vi "TDK电流加载.vi"(5 "all rows":dbl[][](array[numeric]), 6 "停止":bool, 7 "电源台数":dbl=1.0, 8 "循环次数":i32, 9 "error out":errorcluster, 10 "Globalize (0: Single)":u16, 11 "VISA resource name out":refnum<visa-resource-name>) -> (1 "已完成循环次数":i32, 2 "error out 2":errorcluster caption="error out", 3 "VISA resource name out 2":refnum<visa-resource-name>)   [LabVIEW 2021]
uses:
  <instrlib>/TDK-Lambda G Series/TDK-Lambda G Series.lvlib
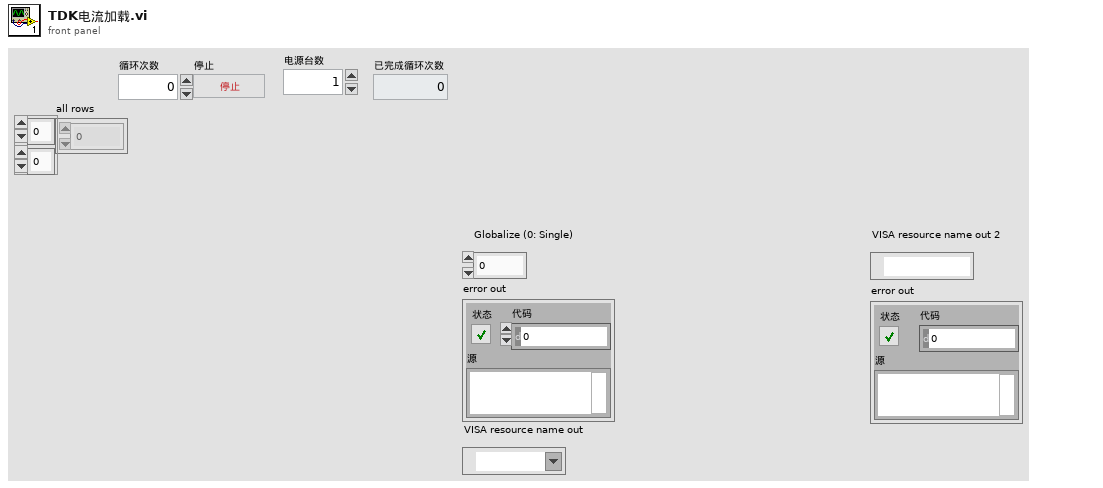
[diagram p1: front panel]
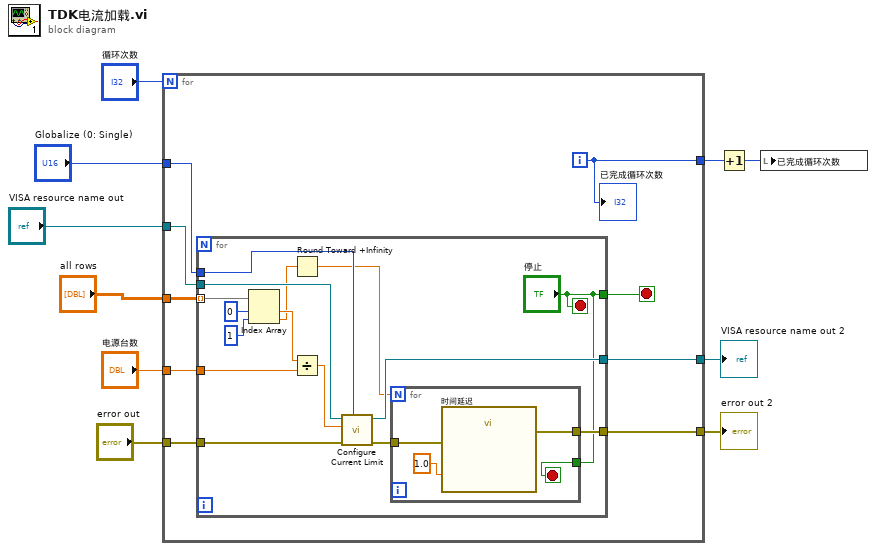
[diagram p0: block diagram]
diagram:
  n1 = for {
    N: "循环次数" -> [_]
    tunnel: "all rows" -> [w17]
    tunnel: "Globalize (0: Single)" -> [w16]
    tunnel: [w15] -> w9
    tunnel: "电源台数" -> [w14]
    tunnel: "error out" -> [w18]
    tunnel: [w11] -> w2
    tunnel: "VISA resource name out" -> [w19]
    tunnel: [w12] -> w3
    i -> [w15]
    stop <- w13 stop-if-true
    n2 = for {
      tunnel: w17 -> [w34] mode=indexing
      tunnel: w19 -> [w31]
      tunnel: w18 -> [w30]
      tunnel: [w28] -> w11
      tunnel: [w27] -> w12
      tunnel: w16 -> [w26]
      tunnel: w14 -> [w23]
      tunnel: ["停止"] -> w13
      stop <- "停止" stop-if-true
      n3 = Index Array(array=w34, index #1=0 ("索引"), index #2=1 ("索引")) -> (element #1=w25:dbl, element #2=w22:dbl)
      n4 = Round Toward +Infinity(x=w22) -> (ceil(x): smallest int >= x=w21:dbl)
      n5 = Divide(x=w25, y=w23) -> (x/y=w24:dbl)
      n6 = call <instrlib>:"Configure Current Limit.vi"("Globalize (0: Single)"=w26, "error in (no error)"=w30, "Current Limit (0A)"=w24, "VISA resource name"=w31) -> ("error out"=w29:errorcluster, "VISA resource name out"=w27:refnum<visa-resource-name>)  [unwired: 6 in]
      n7 = for {
        N: w21 -> [_]
        tunnel: w29 -> [w38]
        tunnel: [w37] -> w28
        tunnel: "停止" -> [w35]
        stop <- w35 stop-if-true
        n8 = call "时间延迟"("error in (no error)"=w38, "Delay Time (s)"=1.0) -> ("error out"=w37:errorcluster)  [unwired: 9 in]
      }
    }
    "已完成循环次数" <- w15
  }
  "VISA resource name out 2" <- w3
  "error out 2" <- w2
  n9 = Increment(x=w9) -> (x+1=w8:i32)
  n10 = local write "已完成循环次数"(w8) -> ()
